vi "initialise.vi"(8 "error in (no error)":errorcluster, 11 "Stimulator090724 in":refnum<class "Stimulator090724Scaffold.lvclass">) -> (0 "error out":errorcluster, 3 "Stimulator090724 out":refnum<class "Stimulator090724Scaffold.lvclass">)   [LabVIEW 2010, in "Stimulator090724Scaffold.lvclass"]
doc: "The dynamic dispatch-version of this VI initalises the plug-in object by allocating and initalising any dynamic resources need."
uses:
  Stimulator090724Scaffold.lvclass
  GenericStimulator/GenericStimulator/GenericStimulator.lvclass
  Stimulator090724Scaffold.lvclass/Stimulator090724Scaffold.ctl
  Clock/GenericClock/GenericClock/GenericClock.lvclass
  common/classes/ErrorController/ErrorController/class_data.vi
  common/classes/ErrorController/ErrorController/ErrorController.lvclass
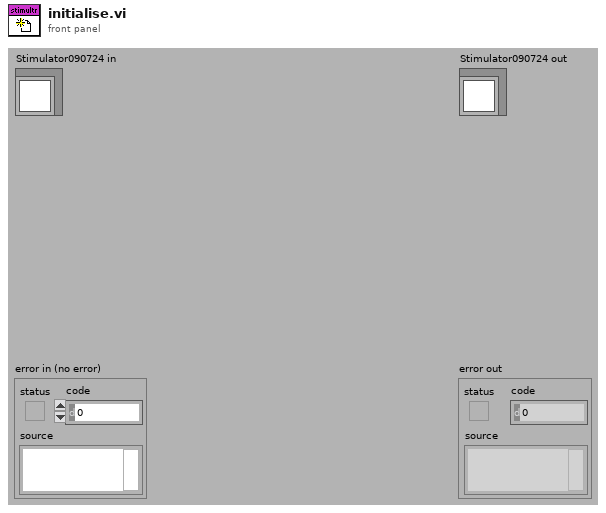
[diagram p1: front panel]
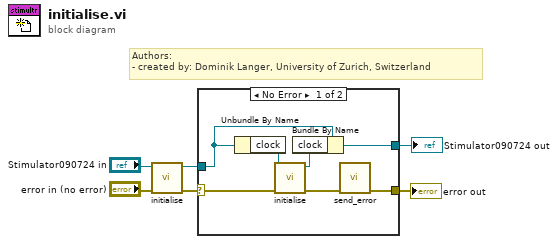
[diagram p0: block diagram]
diagram:
  # "Authors: \n- created by: Dominik Langer, University of Zurich, Switzerland"
  n1 = call-parent "initialise.vi"("error in (no error)"="error in (no error)", "GenericPlugin in"="Stimulator090724 in") -> ("error out"=w4:errorcluster, "GenericPlugin out"=w3:refnum<class "Stimulator090724Scaffold.lvclass">)  [unwired: 8 out]
  n2 = case shown="No Error" w4 {
    selector: w4 -> [w8 w14]
    tunnel: w3 -> [w12 w15]
    tunnel: [w11 w15] -> w2
    tunnel: [w9 w14] -> w1
    frame No Error {
      n3 = Unbundle By Name(w12) -> ("clock"=w7:refnum<class "GenericClock.lvclass">)
      n4 = call-dynamic "initialise.vi"("error in (no error)"=w8, "GenericPlugin in"=w7) -> ("error out"=w10:errorcluster, "GenericPlugin out"=w13:refnum<class "GenericClock.lvclass">)  [unwired: 8 out]
      n5 = Bundle By Name(cluster=w12, "clock"=w13) -> (w11:refnum<class "Stimulator090724Scaffold.lvclass">)
      n6 = call "send_error.vi"("error in (no error)"=w10) -> ("error out"=w9:errorcluster)  [unwired: 10 in]
    }
    frame Error {
    }
  }
  "error out" <- w1
  "Stimulator090724 out" <- w2
